vi "Result Row Color.vi"(8 "error in":errorcluster, 10 "Array":bool[](array[boolean]), 11 "XLS in":refnum<class "XLS.lvclass">=refnum) -> (0 "error out":errorcluster, 3 "XLS out":refnum<class "XLS.lvclass">)   [LabVIEW 2017, in "Report_lib.lvlib" / "XLS.lvclass"]
doc: "This method performs and set color\nrow based on result Boolean Array"
uses:
  XLS.lvclass
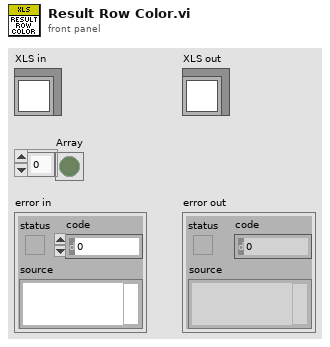
[diagram p1: front panel]
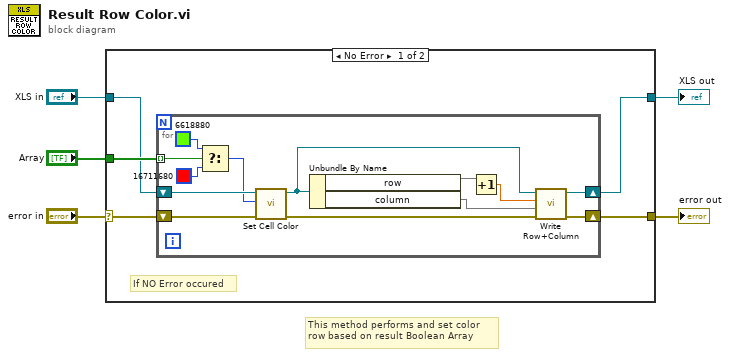
[diagram p0: block diagram]
diagram:
  # "This method performs and set color\nrow based on result Boolean Array"
  n1 = case shown="No Error" "error in" {
    selector: "error in" -> [w9 w25]
    tunnel: [w8 w25] -> w4
    tunnel: [w6 w24] -> w2
    tunnel: "XLS in" -> [w7 w24]
    tunnel: "Array" -> [w10 _]
    frame No Error {
      # "If NO Error occured"
      n2 = for {
        tunnel: w10 -> [w22] mode=indexing
        shift-right: [w13] -> w8
        shift-left: w9 -> [w18]
        shift-right: [w12] -> w6
        shift-left: w7 -> [w23]
        n3 = Select(t=u32 6618880, s=w22, f=u32 16711680) -> (s? t:f=w19:u32)
        n4 = call "Set Cell Color.vi"("error in"=w18, "color"=w19, "XLS in"=w23) -> ("error out"=w14:errorcluster, "XLS out"=w11:refnum<class "XLS.lvclass">)  [unwired: 7 in]
        n5 = Unbundle By Name(w11) -> ("row"=w17, "column"=w15)
        n6 = Increment(x=w17) -> (x+1=w16:dbl)
        n7 = call "Write Row+Column.vi"("error in"=w14, "column"=w15, "row"=w16, "XLS in"=w11) -> ("error out"=w13:errorcluster, "XLS out"=w12:refnum<class "XLS.lvclass">)  [unwired: 6 in]
      }
    }
    frame Error {
    }
  }
  "error out" <- w4
  "XLS out" <- w2
